vi "Error to OK or NG.vi"(11 "error in (no error)":errorcluster) -> (2 "Error source":string, 3 "OK/NG":string)   [LabVIEW 2021]
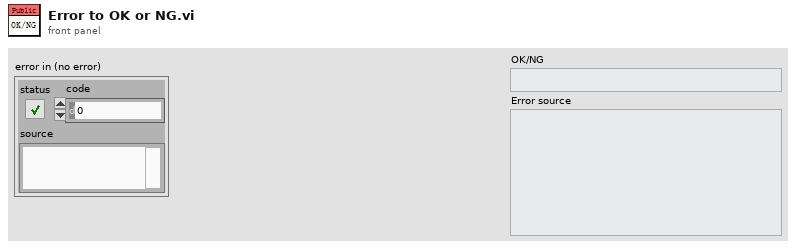
[diagram p1: front panel]
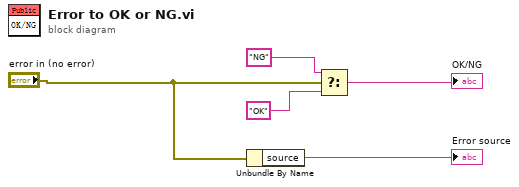
[diagram p0: block diagram]
diagram:
  n1 = Unbundle By Name("error in (no error)") -> ("source"=→"Error source":string)
  n2 = Select(t="NG", s="error in (no error)", f="OK") -> (s? t:f=→"OK/NG":string)
